vi "DB Tools Set Parameter Value.vi"   [LabVIEW 2013, in "NI_Database_API_64.lvlib"]
doc: "Sets the value of the parameter at <B>parameter index</B> in the command or command-recordset. The <B>parameter index</B> can be either the zero-indexed position of the parameter in the command or the name of the parameter. Wire data to the reference input to determine the polymorphic instance to use or manually select the instance."
uses:
  NI_Database_API_64.lvlib
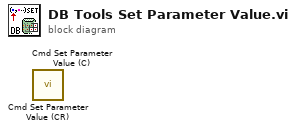
[diagram p0: block diagram]
diagram:
  n1 = call "Cmd Set Parameter Value (CR).vi"() -> ()  [unwired: 8 in, 2 out]
  n2 = call "Cmd Set Parameter Value (C).vi"() -> ()  [unwired: 8 in, 2 out]
